vi "ModStarted.vi"(10 "StartArgs":T1, 11 "DebugTraceHandle":refnum<class "DebugTraceHandle.lvclass">) -> ()   [LabVIEW 2024, in "DebugTraceHandle.lvclass"]
uses:
  DebugTraceHandle.lvclass
  StartArgs.ctl
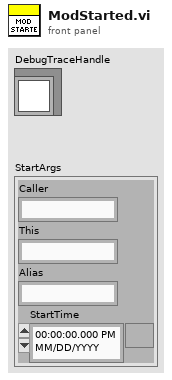
[diagram p1: front panel]
types:
  T1 = typedef "DebugTraceHandle.lvclass/StartArgs.ctl" = cluster{"Caller":string, "This":string, "Alias":string, "StartTime":timestamp}
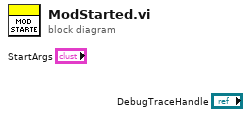
[diagram p0: block diagram]
diagram:
